vi "Global.vi"() -> ()   [LabVIEW 2015]
panel:
  in  "attachment path":path
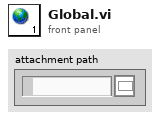
[diagram p1: front panel]
diagram:
